vi "Convert to Big-Endian.vi"(1 "byte":u16(ring)=1 items=["Unsigned Int8"=1, "Unsigned Int16"=2, "Unsigned Int32"=4, "Unsigned Int64"=8], 2 "Input":u8[](array[numeric])) -> (0 "Output":u8[](array[numeric]))   [LabVIEW 2011]
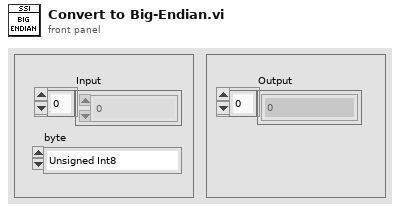
[diagram p1: front panel]
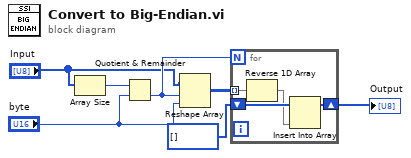
[diagram p0: block diagram]
diagram:
  n1 = Array Size(array="Input") -> (size(s)=w4:i32)
  n2 = Quotient & Remainder(x=w4, y="byte") -> (floor(x/y)=w6:i32)  [unwired: 1 out]
  n3 = Reshape Array("Input", w6, "byte") -> (w5:u8[][])
  n4 = for {
    N: w6 -> [_]
    tunnel: w5 -> [w11] mode=indexing
    shift-right: [w9] -> w3
    shift-left: u8[] [] -> [w10]
    n5 = Reverse 1D Array(array=w11) -> (reversed array=w8:u8[])
    n6 = Insert Into Array(array=w10, new element=w8) -> (w9:u8[])  [unwired: 1 in]
  }
  "Output" <- w3
